vi "Dequeue.vi"(8 "error in":errorcluster) -> (0 "error out":errorcluster, 2 "Data":variant, 3 "State":T1)   [LabVIEW 2018, in "Controller.lvlib"]
uses:
  Controller.lvlib
  ctl/Module - State.ctl
  ctl/Module Queue - Action.ctl
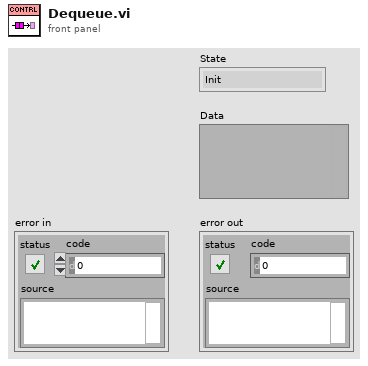
[diagram p1: front panel]
types:
  T1 = typedef "Controller.lvlib/Module - State.ctl" = enum16{"Init", "Idle", "Error", "Close"}
  T2 = typedef "Controller.lvlib/Module Queue - Action.ctl" = enum16{"Create", "Get", "Destroy"}
  T3 = typedef "template.lvlib/Module - Message.ctl" = cluster{"State":T4, "Data":variant}
  T4 = typedef "template.lvlib/Module - State.ctl" = enum16{"Init", "Idle", "Error", "Close"}
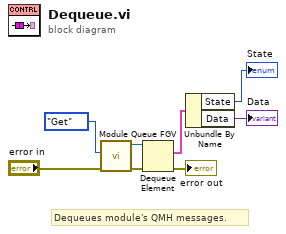
[diagram p0: block diagram]
diagram:
  # "Dequeues module's QMH messages."
  n1 = call "Module Queue FGV.vi"("Error in"="error in", "Action"=Module_Queue_-_Action."Get") -> ("Error out"=w4:errorcluster, "Queue ref"=w3:refnum<queue>)  [unwired: 8 in]
  n2 = Dequeue Element(queue=w3, error in (no error)=w4) -> (element=w6:T3, error out=→"error out":errorcluster)  [unwired: 1 in, 2 out]
  n3 = Unbundle By Name(w6) -> ("State"=→"State":T4, "Data"=→"Data":variant)
